vi "CamAcqu_WaitForTrigger.vi"(10 "Session in":T2, 11 "Image in":T1) -> (1 "Acquisition OK?":bool, 2 "Session Out":T2, 3 "Image  Out":T1)   [LabVIEW 2020]
uses:
  IMAQdx.ctl
  IMAQ Image.ctl
  NI_Vision_Development_Module.lvlib
  NI_Vision_Acquisition_Software.lvlib
panel:
  in  "error in":errorcluster
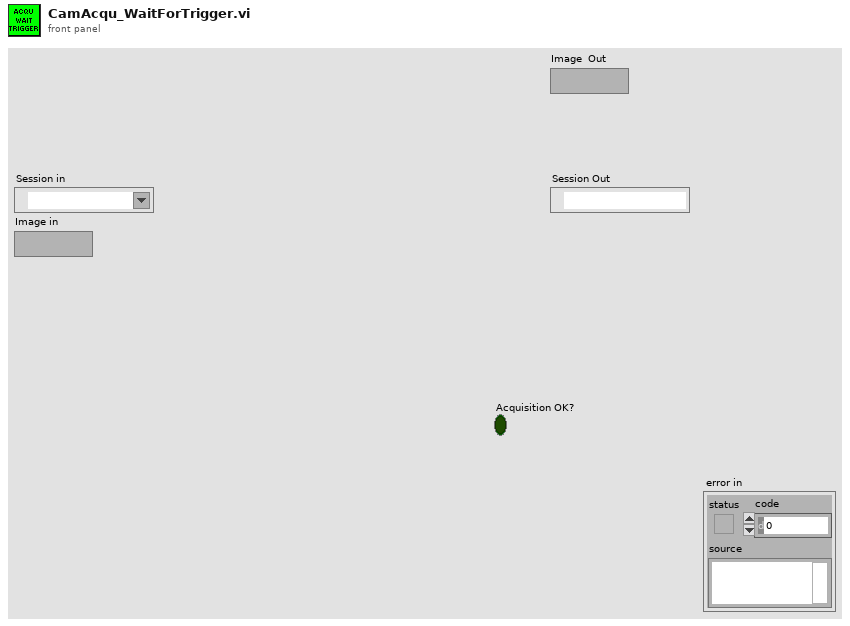
[diagram p1: front panel]
types:
  T1 = typedef "IMAQ Image.ctl" = refnum<image>
  T2 = typedef "IMAQdx.ctl" = refnum<k21>
  T3 = typedef "Image Type" = u32
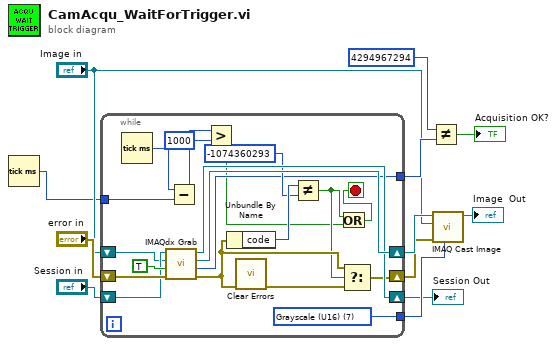
[diagram p0: block diagram]
diagram:
  n1 = Tick Count (ms)() -> (millisecond timer value=w1:u32)
  n2 = while {
    tunnel: [w31] -> w12
    tunnel: [w20] -> w8
    shift-right: [w23] -> w7
    shift-left: "error in" -> [w29]
    shift-right: [w30] -> w11
    shift-left: "Image in" -> [w21]
    shift-right: [w28] -> w3
    shift-left: "Session in" -> [w22]
    tunnel: w1 -> [w18]
    stop <- w13 stop-if-true
    w31 = T3 7 items=["Grayscale (U8)", "Grayscale (I16)", "Grayscale (SGL)", "Complex (CSG)", "RGB (U32)", "HSL (U32)", "RGB (U64)", "Grayscale (U16)"] ("Image Type")
    n3 = Tick Count (ms)() -> (millisecond timer value=w19:u32)
    n4 = call "IMAQdx Grab.vi"("error in"=w29, "Wait for Next Buffer? (Yes)"=TRUE, "Image In"=w21, "Session In"=w22) -> ("error out"=w25:errorcluster, "Buffer Number Out"=w20:u32, "Image Out"=w30:T1, "Session Out"=w28:T2)  [unwired: 4 out]
    n5 = Subtract(x=w19, y=w18) -> (x-y=w17:u32)
    n6 = Greater?(x=w17, y=u32 1000) -> (0:w14:bool)
    n7 = Unbundle By Name(w25) -> ("code"=w27:i32)
    n8 = call "Clear Errors.vi"("error in (no error)"=w25) -> ("error out"=w24:errorcluster)  [unwired: 5 in, 1 out]
    n9 = Not Equal?(x=w27, y=-1074360293 ("code 2")) -> (x != y?=w15:bool)
    n10 = Or(x=w15, y=w14) -> (x .or. y?=w13:bool)
    n11 = Select(t=w25, s=w15, f=w24) -> (s? t:f=w23:errorcluster)
  }
  "Session Out" <- w3
  n12 = Not Equal?(x=u32 4294967294 ("Buffer Number Out"), y=w8) -> (x != y?=→"Acquisition OK?":bool)
  n13 = call "IMAQ Cast Image"("Image Type"=w12, "error in (no error)"=w7, "Image Dst"="Image in", "Image Src"=w11) -> ("Image Dst Out"=→"Image  Out":T1)  [unwired: 6 in, 1 out]
